vi "Run Remote Services.vi"(8 "error in (no error)":errorcluster, 11 "Vecto in":refnum<class "Vecto.lvclass">) -> (0 "error out":errorcluster, 2 "Run Remote Services":bool, 3 "Vecto out":refnum<class "Vecto.lvclass">)   [LabVIEW 2020, in "Vecto.lvlib" / "Vecto.lvclass"]
uses:
  Vecto.lvclass
  Vecto.lvclass/Vecto.ctl
  Node Config/Node Config.lvclass
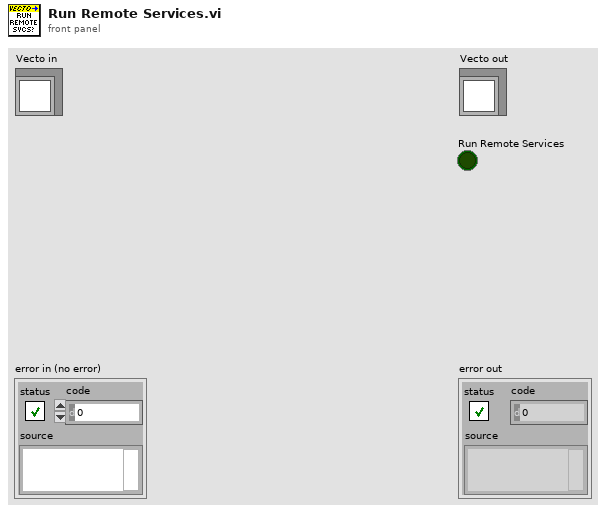
[diagram p1: front panel]
types:
  T1 = typedef "Vecto.lvlib/Discovery Info.ctl" = cluster{"Address":string, "Port":u16, "Interval S":dbl}
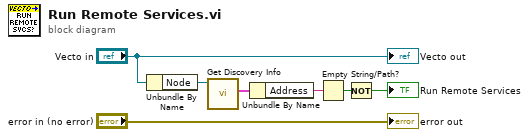
[diagram p0: block diagram]
diagram:
  n1 = Unbundle By Name("Vecto in") -> ("Node"=w6:refnum<class "Node Config.lvclass">)
  n2 = call "Get Discovery Info.vi"("Node in"=w6) -> ("Discovery Info"=w4:T1)  [unwired: 8 in, 2 out]
  n3 = Unbundle By Name(w4) -> ("Address"=w3:string)
  n4 = Empty String/Path?(string/path=w3) -> (empty?=w2:bool)
  n5 = Not(x=w2) -> (.not. x?=→"Run Remote Services":bool)
  "error out" <- "error in (no error)"
  "Vecto out" <- "Vecto in"
